vi "PID FXP Template Multi-Channel PID.vi"(0 "process variable":fxp<+/-,16,5>, 1 "reset?":bool, 12 "configuration":T1={"PID gains"={"proportional gain (Kc)"=1.0, "integral gain (Kc*Ts/Ti)"=0.01171875, "derivative gain (Kc*Td/Ts)"=0.0}, "output range"={"output high"=32767.0, "output low"=-32768.0}, "setpoint"=0.0, "channel index"=0} {"PID gains"."proportional gain (Kc)" format="%.11g"; "PID gains"."integral gain (Kc*Ts/Ti)" format="%.11g"; "PID gains"."derivative gain (Kc*Td/Ts)" format="%.11g"}) -> (4 "output":fxp<+/-,16,16>, 8 "channel index":u16)   [LabVIEW 2017]
doc: "On an FPGA target, implements an integer PID algorithm for PID applications with high-speed control and/or high channel count that require an efficient algorithm. You can use this Express VI with single-channel or multi-channel configurations. The PID algorithm features control action range and uses the integrator anti-windup calculation to limit the effect of the integral action during transients. The PID algorithm also features bumpless controller output for PID gain changes.\n--------------------------------------------------------\n\nThis Express VI is configured as follows:\n\nNumber of channels = 1\nProportional gain (Kc) = 1\nIntegral time (Ti) = 10mmin\nDerivative time (Td) = 0min\nSampling time (Ts) = 1s\nProportional gain (scaled) (Kc * 2^8) = 256\nIntegral gain (scaled) ([Kc*Ts]/[Ti*60] * 2^8) = 427\nDerivative gain (scaled) ([Kc*Td*60]/[Ts] * 2^8) = 0\nOutput range high = 32767\nOutput range low = -32768\nInitial setpoint = 0"
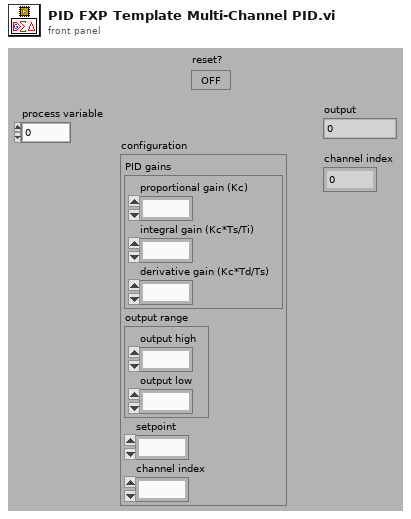
[diagram p1: front panel]
types:
  T1 = cluster{"PID gains":cluster{"proportional gain (Kc)":fxp<+/-,16,8>, "integral gain (Kc*Ts/Ti)":fxp<+/-,16,8>, "derivative gain (Kc*Td/Ts)":fxp<+/-,16,8>}, "output range":cluster{"output high":fxp<+/-,16,16>, "output low":fxp<+/-,16,16>}, "setpoint":fxp<+/-,16,16>, "channel index":u16}
  T2 = cluster{"PID gains (x 2^8)":cluster{"proportional gain (Kc)":i16, "integral gain (Kc*Ts/Ti)":i16, "derivative gain (Kc*Td/Ts)":i16}, "output range":cluster{"output high":i16, "output low":i16}, "setpoint":i16, "channel index":u16}
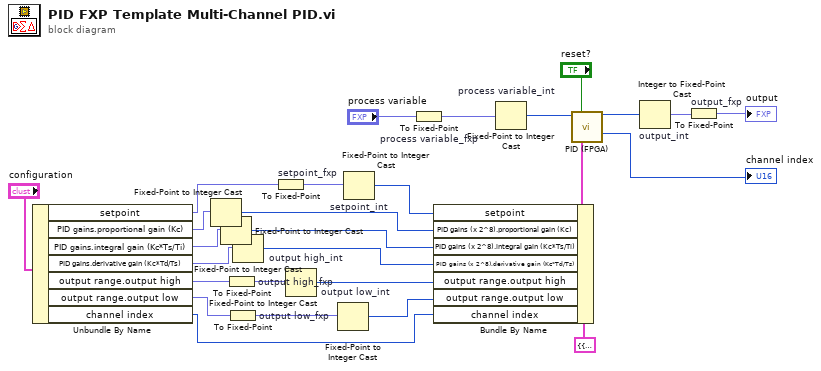
[diagram p0: block diagram]
diagram:
  n1 = Unbundle By Name("configuration") -> ("setpoint"=w25:fxp<+/-,16,16>, "PID gains.proportional gain (Kc)"=w8:fxp<+/-,16,8>, "PID gains.integral gain (Kc*Ts/Ti)"=w7:fxp<+/-,16,8>, "PID gains.derivative gain (Kc*Td/Ts)"=w6:fxp<+/-,16,8>, "output range.output high"=w5:fxp<+/-,16,16>, "output range.output low"=w4:fxp<+/-,16,16>, "channel index"=w3:u16)
  n2 = Fixed-Point to Integer Cast(1:w8) -> (0:w15:i16)
  n3 = Fixed-Point to Integer Cast(1:w7) -> (0:w14:i16)
  n4 = To Fixed-Point "output high_fxp"(number=w5) -> (fixed-point=w12:fxp<+/-,16,16>)  [unwired: 1 out]
  n5 = To Fixed-Point "output low_fxp"(number=w4) -> (fixed-point=w10:fxp<+/-,16,16>)  [unwired: 1 out]
  n6 = Fixed-Point to Integer Cast(1:w6) -> (0:w13:i16)
  n7 = To Fixed-Point "setpoint_fxp"(number=w25) -> (fixed-point=w16:fxp<+/-,16,16>)  [unwired: 1 out]
  n8 = Fixed-Point to Integer Cast "output high_int"(1:w12) -> (0:w11:i16)
  n9 = Fixed-Point to Integer Cast "output low_int"(1:w10) -> (0:w9:i16)
  n10 = Fixed-Point to Integer Cast "setpoint_int"(1:w16) -> (0:w17:i16)
  n11 = To Fixed-Point "process variable_fxp"(number="process variable") -> (fixed-point=w20:fxp<+/-,16,5>)  [unwired: 1 out]
  n12 = Bundle By Name(cluster=T2 {"PID gains (x 2^8)"={"proportional gain (Kc)"=256, "integral gain (Kc*Ts/Ti)"=427, "derivative gain (Kc*Td/Ts)"=0}, "output range"={"output high"=32767, "output low"=-32768}, "setpoint"=0, "channel index"=0} ("configuration"), "setpoint"=w17, "PID gains (x 2^8).proportional gain (Kc)"=w15, "PID gains (x 2^8).integral gain (Kc*Ts/Ti)"=w14, "PID gains (x 2^8).derivative gain (Kc*Td/Ts)"=w13, "output range.output high"=w11, "output range.output low"=w9, "channel index"=w3) -> (w2:T2)
  n13 = Fixed-Point to Integer Cast "process variable_int"(1:w20) -> (0:w21:i16)
  n14 = call "PID (FPGA).vi"("process variable"=w21, "reset?"="reset?", "configuration"=w2) -> ("output"=w19:i16, "channel index"=→"channel index":u16)  [unwired: 11 in]
  n15 = Integer to Fixed-Point Cast "output_int"(integer=w19) -> (fixed-point=w18:fxp<+/-,16,16>)  [unwired: 1 in]
  n16 = To Fixed-Point "output_fxp"(number=w18) -> (fixed-point=→"output":fxp<+/-,16,16>)  [unwired: 1 out]
